vi "Scan lvclass.vi"(8 "error in (no error)":errorcluster, 10 "App Refnum":refnum<vi>, 11 "Path":path) -> (0 "error out":errorcluster, 1 "Public Events Paths":path[](array[path]), 2 "Foreground Color":u32(colorbox), 3 "Public Events":string[](array[string]))   [LabVIEW 2016, in "LV Object Event Registration Node.xnode"]
uses:
  LV Object Event Registration Node.xnode
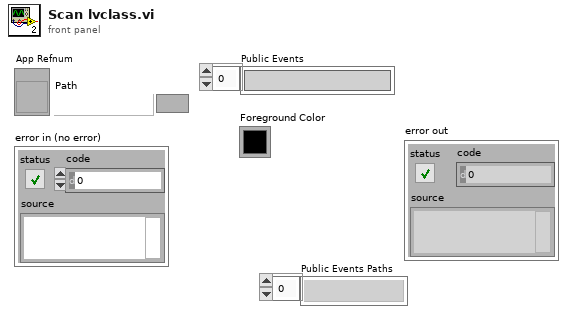
[diagram p1: front panel]
types:
  T1 = cluster{"Foreground Color":u32, "Background Color":u32, "Fill Pattern":cluster{"Row 0":u8, "Row 1":u8, "Row 2":u8, "Row 3":u8, "Row 4":u8, "Row 5":u8, "Row 6":u8, "Row 7":u8}, "Width":i16, "Mode":enum16{"Copy", "Or", "Exclusive Or", "Bit Clear", "Not Copy", "Not Or", "Nor Exclusive Or", "Not Bit Clear"}, "Style":enum32{"Solid", "Dash", "Dot", "Dash Dot", "Dash Dot Dot"}, "Fill Rule":enum32{"Even Odd", "Winding"}, "End Caps":enum32{"Default", "Flat"}}[]
  T2 = cluster{"Foreground Color":u32, "Background Color":u32, "Fill Pattern":cluster{"Row 0":u8, "Row 1":u8, "Row 2":u8, "Row 3":u8, "Row 4":u8, "Row 5":u8, "Row 6":u8, "Row 7":u8}, "Width":i16, "Mode":enum16{"Copy", "Or", "Exclusive Or", "Bit Clear", "Not Copy", "Not Or", "Nor Exclusive Or", "Not Bit Clear"}, "Style":enum32{"Solid", "Dash", "Dot", "Dash Dot", "Dash Dot Dot"}, "Fill Rule":enum32{"Even Odd", "Winding"}, "End Caps":enum32{"Default", "Flat"}}
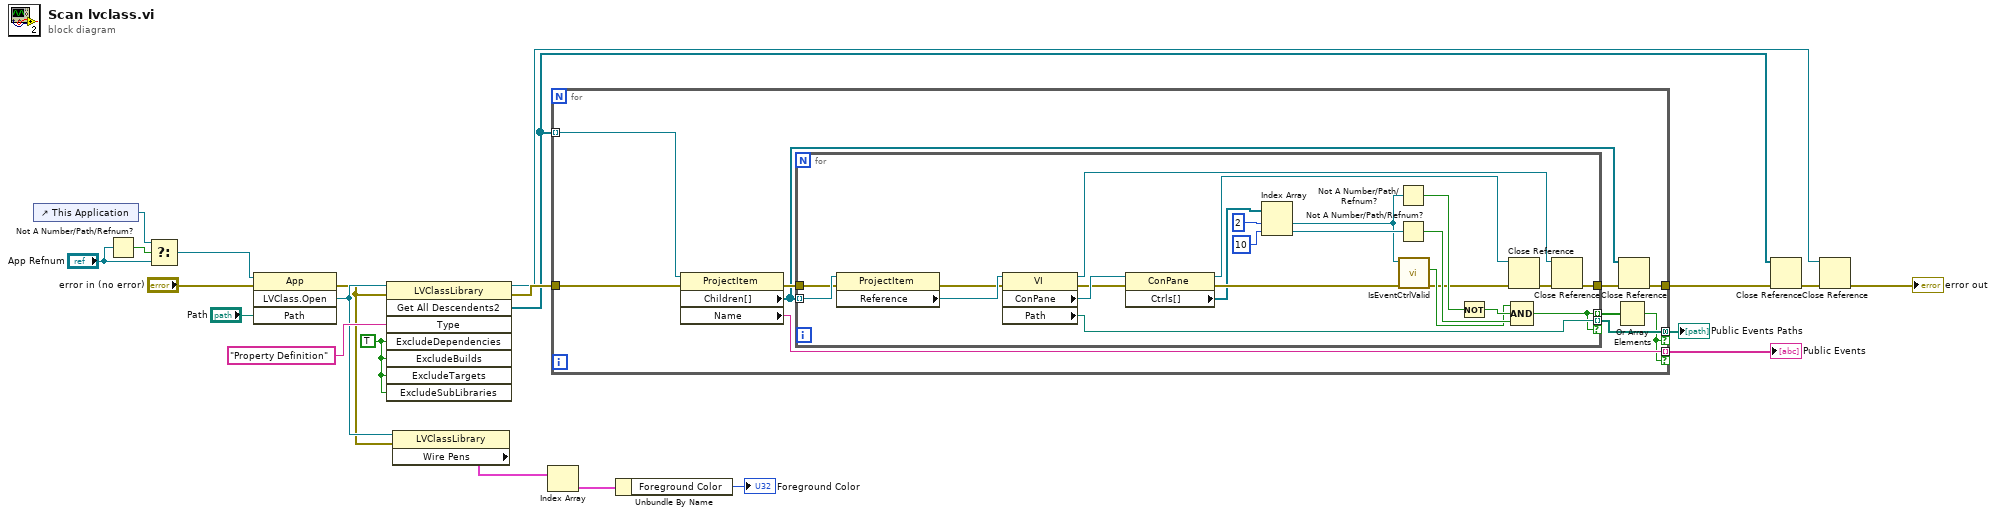
[diagram p0: block diagram]
diagram:
  w17 = TRUE ("ExcludeDependencies")
  n1 = control-ref of="This Application"() -> (w11:refnum<vi>)
  n2 = Not A Number/Path/Refnum?(number/path/refnum="App Refnum") -> (NaN/Path/Refnum?=w13:bool)
  n3 = Select(t=w11, s=w13, f="App Refnum") -> (s? t:f=w10:refnum<vi>)
  n4 = invoke class="App" method="LVClass.Open"(reference=w10, error in="error in (no error)", "Path"="Path") -> (error out=w8:errorcluster, "LVClass.Open"=w15:refnum<vi>)  [unwired: 1 in, 2 out]
  n5 = invoke class="LVClassLibrary" method="Get All Descendents2"(reference=w15, error in=w8, "Type"="Property Definition", "ExcludeDependencies"=w17, "ExcludeBuilds"=w17, "ExcludeTargets"=w17, "ExcludeSubLibraries"=w17) -> (reference out=w4:refnum<vi>, error out=w7:errorcluster, "Get All Descendents2"=w6:refnum<vi>[])  [unwired: 1 in, 5 out]
  n6 = property class="LVClassLibrary"(reference=w15, error in=w8) -> ("Wire Pens"=w18:T1)  [unwired: 2 out]
  n7 = Index Array(array=w18) -> (element=w19:T2)  [unwired: 1 in]
  n8 = for {
    tunnel: w6 -> [w31] mode=indexing
    tunnel: [w29] -> w21 mode=indexing if=w22
    tunnel: w7 -> [w28]
    tunnel: [w24] -> w5
    tunnel: [w23] -> w1 mode=concatenating if=w22
    n9 = property class="ProjectItem"(reference=w31, error in=w28) -> (error out=w27:errorcluster, "Children[]"=w26:refnum<vi>[], "Name"=w29:string)  [unwired: 1 out]
    n10 = for {
      tunnel: w26 -> [w54] mode=indexing
      tunnel: [w32] -> w30 mode=indexing
      tunnel: [w34] -> w25
      tunnel: w27 -> [w42]
      tunnel: [w33] -> w23 mode=indexing if=w32
      n11 = property class="ProjectItem"(reference=w54, error in=w42) -> (error out=w41:errorcluster, "Reference"=w52:refnum<vi>)  [unwired: 1 out]
      n12 = property class="VI"(reference=w52, error in=w41) -> (reference out=w35:refnum<vi>, error out=w40:errorcluster, "ConPane"=w53:refnum<vi>, "Path"=w33:path)
      n13 = property class="ConPane"(reference=w53, error in=w40) -> (reference out=w37:refnum<vi>, error out=w45:errorcluster, "Ctrls[]"=w38:refnum<vi>[])
      n14 = Index Array(array=w38, index #1=2 ("index"), index #2=10 ("index")) -> (element #1=w43:refnum<vi>, element #2=w49:refnum<vi>)
      n15 = Not A Number/Path/Refnum?(number/path/refnum=w43) -> (NaN/Path/Refnum?=w48:bool)
      n16 = Not A Number/Path/Refnum?(number/path/refnum=w49) -> (NaN/Path/Refnum?=w46:bool)
      n17 = call "IsEventCtrlValid.vi"("error in (no error)"=w45, "Control in"=w43) -> ("error out"=w39:errorcluster, "Boolean"=w44:bool)  [unwired: 8 in]
      n18 = Not(x=w48) -> (.not. x?=w47:bool)
      n19 = Close Reference(reference=w37, error in (no error)=w39) -> (error out=w36:errorcluster)
      n20 = Compound Arithmetic op=AND(w44, w47, w46) -> (w32:bool)
      n21 = Close Reference(reference=w35, error in (no error)=w36) -> (error out=w34:errorcluster)
    }
    n22 = Or Array Elements(Boolean array=w30) -> (logical OR=w22:bool)
    n23 = Close Reference(reference=w26, error in (no error)=w25) -> (error out=w24:errorcluster)
  }
  "Public Events" <- w21
  "Public Events Paths" <- w1
  n24 = Unbundle By Name(w19) -> ("Foreground Color"=→"Foreground Color":u32)
  n25 = Close Reference(reference=w6, error in (no error)=w5) -> (error out=w3:errorcluster)
  n26 = Close Reference(reference=w4, error in (no error)=w3) -> (error out=→"error out":errorcluster)
